vi "Update State.vi"(8 "error in (no error)":errorcluster, 11 "UniStableShutter in":refnum<class "UniStableShutter.lvclass">) -> (0 "error out":errorcluster, 3 "UniStableShutter out":refnum<class "UniStableShutter.lvclass">)   [LabVIEW 2016, in "UniStableShutter.lvclass"]
uses:
  UniStableShutter.lvclass
  Controls/Shutter States.ctl
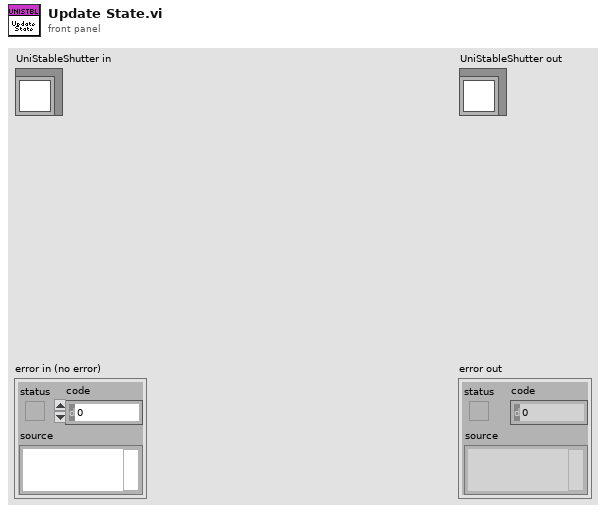
[diagram p1: front panel]
types:
  T1 = typedef "Shutter States.ctl" = enum16{"Open", "Close", "Wait", "Off", "Arm", "Idle"}
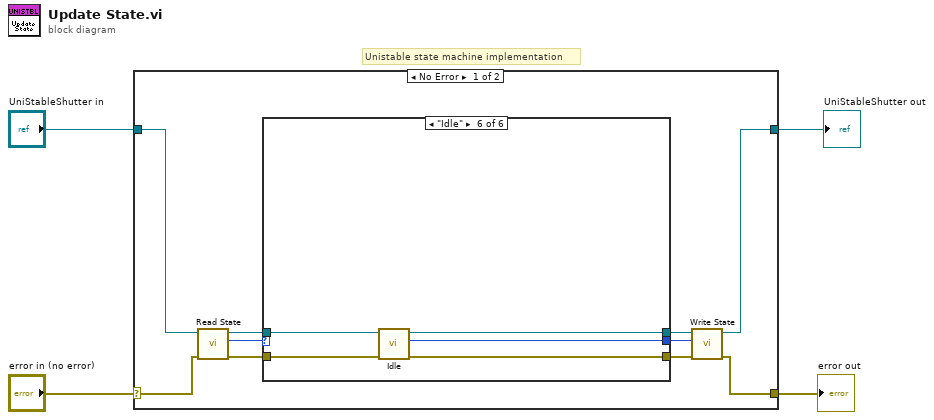
[diagram p0: block diagram]
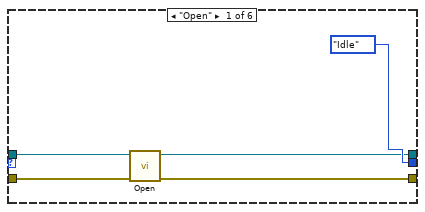
[diagram p2: hidden frame]
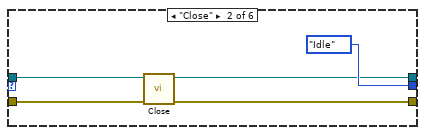
[diagram p3: hidden frame]
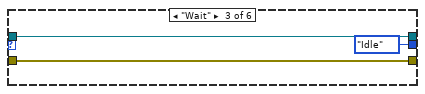
[diagram p4: hidden frame]
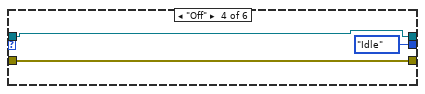
[diagram p5: hidden frame]
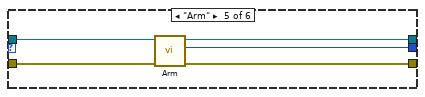
[diagram p6: hidden frame]
diagram:
  # "Unistable state machine implementation"
  n1 = case shown="No Error" "error in (no error)" {
    selector: "error in (no error)" -> [w13 w42]
    tunnel: [w6 w42] -> w4
    tunnel: [w7 w41] -> w3
    tunnel: "UniStableShutter in" -> [w14 w41]
    frame No Error {
      n2 = call-dynamic "Read State.vi"("error in (no error)"=w13, "Shutter in"=w14) -> ("error out"=w11:errorcluster, "State"=w5:T1, "Shutter out"=w12:refnum<class "UniStableShutter.lvclass">)  [unwired: 7 in]
      n3 = case shown="\"Idle\"" w5 {
        tunnel: w12 -> [w18 w23 w26 w28 w35 w40]
        tunnel: w11 -> [w17 w22 w27 w30 w34 w36]
        tunnel: [w15 w20 w26 w28 w31 w39] -> w10
        tunnel: [Shutter_States."Idle" ("Set") Shutter_States."Idle" ("Set") Shutter_States."Idle" ("Set") Shutter_States."Idle" ("Set") w32 w38] -> w9
        tunnel: [w16 w21 w27 w30 w33 w37] -> w8
        frame "Open" {
          n4 = call-dynamic "Open.vi"("error in (no error)"=w17, "UniStableShutter in"=w18) -> ("error out"=w16:errorcluster, "UniStableShutter out"=w15:refnum<class "UniStableShutter.lvclass">)  [unwired: 8 in]
        }
        frame "Close" {
          n5 = call-dynamic "Close.vi"("error in (no error)"=w22, "UniStableShutter in"=w23) -> ("error out"=w21:errorcluster, "UniStableShutter out"=w20:refnum<class "UniStableShutter.lvclass">)  [unwired: 8 in]
        }
        frame "Wait" {
        }
        frame "Off" {
        }
        frame "Arm" {
          n6 = call-dynamic "Arm.vi"("error in (no error)"=w34, "Shutter in"=w35) -> ("error out"=w33:errorcluster, "State"=w32:T1, "Shutter out"=w31:refnum<class "UniStableShutter.lvclass">)  [unwired: 7 in]
        }
        frame "Idle" {
          n7 = call-dynamic "Idle.vi"("error in (no error)"=w36, "Shutter in"=w40) -> ("error out"=w37:errorcluster, "State"=w38:T1, "Shutter out"=w39:refnum<class "UniStableShutter.lvclass">)  [unwired: 7 in]
        }
      }
      n8 = call-dynamic "Write State.vi"("error in (no error)"=w8, "Set"=w9, "Shutter in"=w10) -> ("error out"=w6:errorcluster, "Shutter out"=w7:refnum<class "UniStableShutter.lvclass">)  [unwired: 7 in]
    }
    frame Error {
    }
  }
  "error out" <- w4
  "UniStableShutter out" <- w3
